vi "Get Pos Impl.vi"(8 "error in (no error)":errorcluster, 11 "Newport ESP301 Stage in":refnum<class "Newport ESP301 Stage.lvclass">) -> (0 "error out":errorcluster, 2 "Stage Position":T1, 3 "Newport ESP301 Stage out":refnum<class "Newport ESP301 Stage.lvclass">)   [LabVIEW 2023, in "Newport ESP301 Stage.lvlib" / "Newport ESP301 Stage.lvclass"]
uses:
  Newport ESP301 Stage.lvclass
  Newport ESP301 Stage.lvclass/Newport ESP301 Stage.ctl
  Resources/Type Defs/Stage Position.ctl
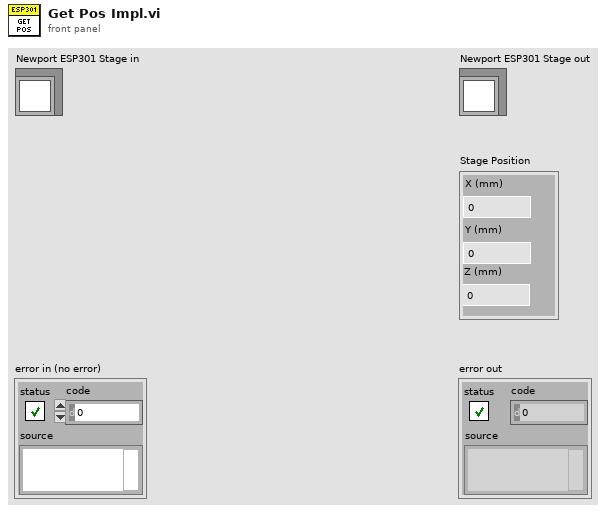
[diagram p1: front panel]
types:
  T1 = typedef "Stage Position.ctl" = cluster{"X (mm)":dbl, "Y (mm)":dbl, "Z (mm)":dbl}
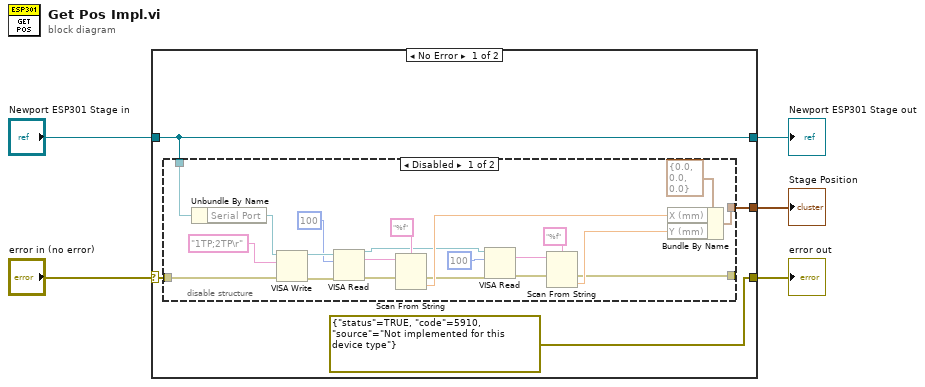
[diagram p0: block diagram]
diagram:
  n1 = case shown="No Error" "error in (no error)" {
    selector: "error in (no error)" -> [w6 w31]
    tunnel: "Newport ESP301 Stage in" -> [w9 w32]
    tunnel: [errorcluster {"status"=TRUE, "code"=5910, "source"="Not implemented for this device type"} ("error IO") w31] -> w3
    tunnel: [w9 w32] -> w2
    tunnel: [w8 _] -> w1
    frame No Error {
      n2 = disable-structure shown="Disabled" {
        disable-tunnel: w9 -> [w28 _]
        disable-tunnel: [w23 _] -> w8
        disable-tunnel: w6 -> [w11 _]
        disable-tunnel: [w10 _] -> _
        frame Disabled {
          n3 = Unbundle By Name(w28) -> ("Serial Port"=w29:refnum<visa-resource-name>)
          n4 = VISA Write(VISA resource name=w29, write buffer="1TP;2TP\r" ("true string"), error in (no error)=w11) -> (VISA resource name out=w26:refnum<visa-resource-name>, error out=w27:errorcluster)  [unwired: 1 out]
          n5 = VISA Read(VISA resource name=w26, byte count=u32 100, error in (no error)=w27) -> (VISA resource name out=w12:refnum<visa-resource-name>, read buffer=w21:string, error out=w22:errorcluster)  [unwired: 1 out]
          n6 = Scan From String(format string="%f", input string=w21, error in=w22) -> (error out=w15:errorcluster, output 1=w19:dbl)  [unwired: 2 in, 2 out]
          n7 = VISA Read(VISA resource name=w12, byte count=u32 100, error in (no error)=w15) -> (read buffer=w17:string, error out=w14:errorcluster)  [unwired: 2 out]
          n8 = Scan From String(format string="%f", input string=w17, error in=w14) -> (error out=w10:errorcluster, output 1=w13:dbl)  [unwired: 2 in, 2 out]
          n9 = Bundle By Name(cluster=T1 {"X (mm)"=0.0, "Y (mm)"=0.0, "Z (mm)"=0.0} ("Stage Position 2"), "X (mm)"=w19, "Y (mm)"=w13) -> (w23:T1)
        }
        frame Enabled {
        }
      }
    }
    frame Error {
    }
  }
  "error out" <- w3
  "Newport ESP301 Stage out" <- w2
  "Stage Position" <- w1
